vi "Handle Click on Tree Item.vi"(5 "Button":u16, 7 "PlatMods":T1, 8 "error in (no error)":errorcluster, 9 "Mods":cluster{"Double Click":bool, "Menu Key":bool}, 10 "Coords":T2, 11 "Test Executive Explorer in":refnum<class "Test Executive Explorer.lvclass">) -> (0 "error out":errorcluster, 3 "Test Executive Explorer out":refnum<class "Test Executive Explorer.lvclass">)   [LabVIEW 2019, in "Test Executive Explorer.lvclass"]
doc: "<RequiredOverrideReason>Implement the response to the user left clicking on the tree.</RequiredOverrideReason>"
uses:
  <vilib>/gpm_packages/@cs/Test-executive-builder/Example/Application/Test Executive Explorer/Test Executive Explorer/Test Executive Explorer.lvclass
  C:/Program Files/National Instruments/LabVIEW 2019/vi.lib/gpm_packages/@cs/file-explorer-extension/Source/File Explorer/File Explorer/File Explorer.lvclass
  <vilib>/Utility/miscctls.llb/LVPoint32TypeDef.ctl
  <vilib>/gpm_packages/@cs/file-explorer-extension/Source/File Explorer/File Explorer/File Explorer.lvclass/File Explorer.ctl
  <vilib>/gpm_packages/@cs/file-explorer-extension/Source/File Explorer/File Explorer/File Explorer.lvclass
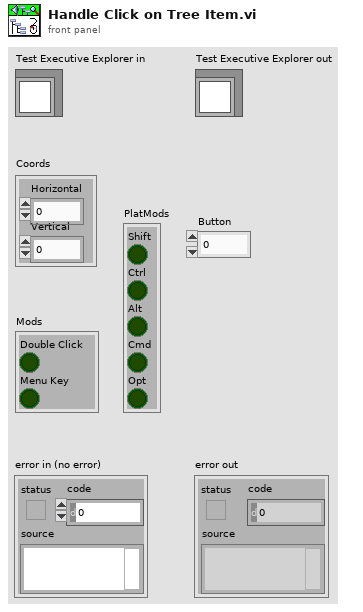
[diagram p1: front panel]
types:
  T1 = cluster{"Shift":bool, "Ctrl":bool, "Alt":bool, "Cmd":bool, "Opt":bool}
  T2 = typedef "LVPoint32TypeDef.ctl" = cluster{"Horizontal":i32, "Vertical":i32}
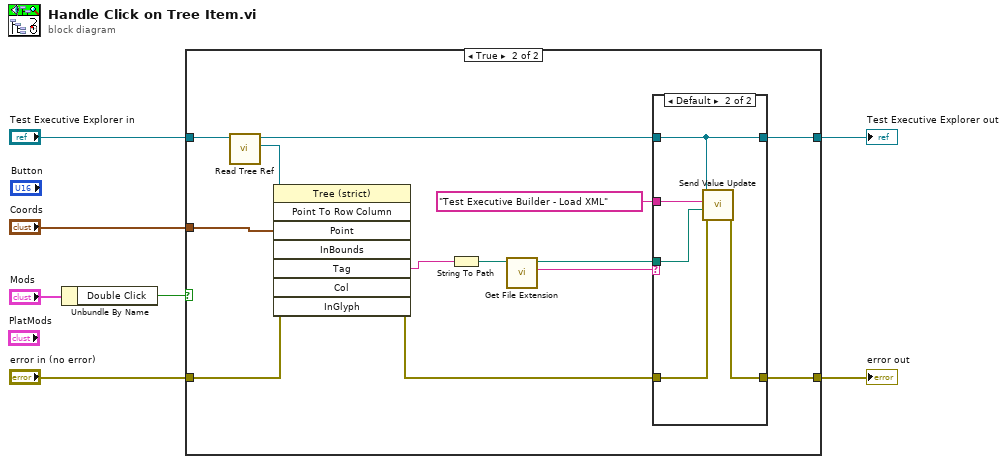
[diagram p0: block diagram]
diagram:
  n1 = Unbundle By Name("Mods") -> ("Double Click"=w1:bool)
  n2 = case shown="True" w1 {
    tunnel: "Test Executive Explorer in" -> [w9 w15]
    tunnel: [w9 w14] -> w5
    tunnel: "error in (no error)" -> [w8 w13]
    tunnel: [w8 w12] -> w3
    tunnel: "Coords" -> [_ w11]
    frame False {
    }
    frame True {
      n3 = call <vilib>:"Read Tree Ref.vi"("File Explorer in"=w15) -> ("Tree Ref"=w10:refnum<vi>, "File Explorer out"=w22:refnum<class "Test Executive Explorer.lvclass">)  [unwired: 8 in, 1 out]
      n4 = invoke class="Tree (strict)" method="Point To Row Column"(reference=w10, error in=w13, "Point"=w11) -> (error out=w19:errorcluster, "Tag"=w17:string)  [unwired: 5 in, 6 out]
      n5 = String To Path(string=w17) -> (path=w21:path)
      n6 = call <vilib>:"Get File Extension.vi"("file"=w21) -> ("lowercase file extension"=w16:string, "dup file"=w18:path)  [unwired: 6 in, 3 out]
      n7 = case shown="Default" w16 {
        tunnel: w22 -> [w23 w25]
        tunnel: "Test Executive Builder - Load XML" ("Datum Name") -> [_ w29]
        tunnel: w19 -> [w24 w28]
        tunnel: [w24 w27] -> w12
        tunnel: w18 -> [_ w26]
        tunnel: [w23 w25] -> w14
        frame "" {
        }
        frame Default {
          n8 = call-dynamic "Send Value Update.vi"("error in (no error)"=w28, "Value"=w26, "Datum Name"=w29, "IViewable in"=w25) -> ("error out"=w27:errorcluster)  [unwired: 7 in]
        }
      }
    }
  }
  "error out" <- w3
  "Test Executive Explorer out" <- w5
